vi "Lockin.DAQ.DAQmx Read.vi"(0 "Refnum in":refnum<k21>, 5 "number of samples per channel":i32, 9 "timeout":dbl, 11 "error in (no error)":errorcluster, 12 "ID in":i32) -> (4 "Refnum out":refnum<k21>, 6 "data":waveform(dbl)[](array[waveform]), 14 "ID out":i32, 15 "error out":errorcluster)   [LabVIEW 2019, in "Instrument.DAQ.lvclass"]
uses:
  Instrument.DAQ.lvclass
  <vilib>/DAQmx/read.llb/DAQmx Read (Analog 1D Wfm NChan NSamp).vi
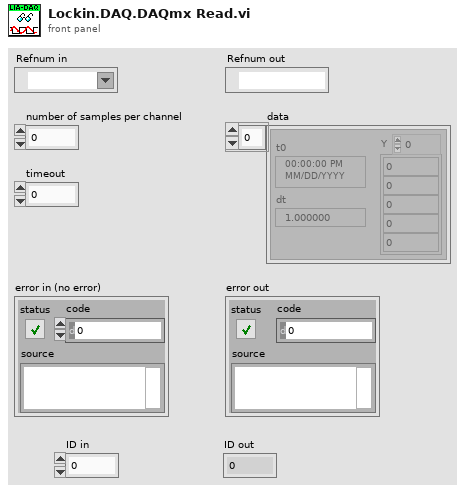
[diagram p1: front panel]
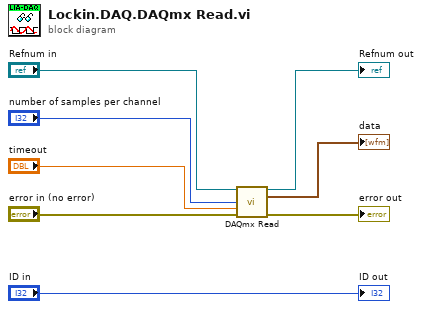
[diagram p0: block diagram]
diagram:
  n1 = call-poly <vilib>:"DAQmx Read.vi"("task/channels in"="Refnum in", "number of samples per channel"="number of samples per channel", "timeout"="timeout", "error in"="error in (no error)") -> ("task out"=→"Refnum out":refnum<k21>, "data"=→"data":waveform(dbl)[], "error out"=→"error out":errorcluster)  [unwired: 9 in]
  "ID out" <- "ID in"
